vi "DIO64 Sequence.vi"(0 "DIO64Addr (0)":u16, 1 "RepRate (Hz)":dbl, 3 "Config Control":T1={"flags"=enum."unused", "clock control"=enum."external", "start trigger"={"source"=enum."external", "type"=enum."edge", "sense"=enum."rising"}, "stop trigger"={"source"=enum."output FIFO", "type"=enum."level", "sense"=enum."falling"}, "DAQ clock modulo"=0, "repetitions"=0, "#transitions"=0} {"#transitions" format="%.0x"; "repetitions" format="%.0x"; "DAQ clock modulo" format="%.0x"}, 5 "Time Array (ms)":dbl[](array[numeric])=[0.0, 1.0, 2.1658, 2.4158, 2.5658, 2.5757999999999996, 2.7057999999999995, 2.7157999999999993, 3.1699999999999995, 3.1913999999999993, 3.2021999999999995, 3.2031999999999994, 3.2226999999999992, 3.223699999999999, 4.223699999999999] caption="Time of step .. (ms)", 7 "Set DIO line ..":bool[][](array[boolean])=[[FALSE, FALSE, FALSE, FALSE, FALSE, FALSE, FALSE, FALSE, FALSE, FALSE, FALSE, FALSE, FALSE, FALSE, FALSE, FALSE], [FALSE, FALSE, FALSE, FALSE, FALSE, FALSE, FALSE, FALSE, FALSE, FALSE, FALSE, FALSE, FALSE, FALSE, FALSE, FALSE], [FALSE, FALSE, FALSE, FALSE, FALSE, FALSE, TRUE, FALSE, FALSE, FALSE, FALSE, FALSE, FALSE, FALSE, FALSE, FALSE], [FALSE, FALSE, FALSE, FALSE, FALSE, FALSE, FALSE, FALSE, FALSE, FALSE, FALSE, FALSE, FALSE, FALSE, FALSE, FALSE], [FALSE, FALSE, FALSE, FALSE, TRUE, FALSE, FALSE, FALSE, FALSE, FALSE, FALSE, FALSE, FALSE, FALSE, FALSE, FALSE], [FALSE, FALSE, FALSE, FALSE, FALSE, FALSE, FALSE, FALSE, FALSE, FALSE, FALSE, FALSE, FALSE, FALSE, FALSE, FALSE], [FALSE, FALSE, FALSE, FALSE, FALSE, TRUE, FALSE, FALSE, FALSE, FALSE, FALSE, FALSE, FALSE, FALSE, FALSE, FALSE], [FALSE, FALSE, FALSE, FALSE, FALSE, FALSE, FALSE, FALSE, FALSE, FALSE, FALSE, FALSE, FALSE, FALSE, FALSE, FALSE], [FALSE, FALSE, FALSE, FALSE, FALSE, FALSE, FALSE, FALSE, FALSE, TRUE, FALSE, FALSE, FALSE, FALSE, FALSE, FALSE], [FALSE, FALSE, FALSE, FALSE, FALSE, FALSE, FALSE, FALSE, FALSE, FALSE, TRUE, FALSE, FALSE, FALSE, FALSE, FALSE], [FALSE, FALSE, FALSE, TRUE, FALSE, FALSE, FALSE, FALSE, FALSE, FALSE, FALSE, FALSE, FALSE, FALSE, FALSE, FALSE], [FALSE, FALSE, FALSE, FALSE, FALSE, FALSE, FALSE, FALSE, FALSE, FALSE, FALSE, FALSE, FALSE, FALSE, FALSE, FALSE], [FALSE, FALSE, FALSE, FALSE, FALSE, FALSE, FALSE, TRUE, FALSE, FALSE, FALSE, FALSE, FALSE, FALSE, FALSE, FALSE], [FALSE, FALSE, FALSE, FALSE, FALSE, FALSE, FALSE, FALSE, FALSE, FALSE, FALSE, FALSE, FALSE, FALSE, FALSE, FALSE]] caption="Set DIO lines in step ..", 9 "output cluster":cluster{bool[][], bool[][], bool[][], bool[][]}, 11 "error in":errorcluster={"status"=FALSE, "code"=0, "source"="DIO64 Out Stop"}) -> (15 "error out":errorcluster={"status"=FALSE, "code"=0, "source"="DIO64 Out Stop"})   [LabVIEW 2012]
doc: "Sets the DIO-Board to - \"Continous Mode\" and\n - External Triggering (Edge, rising)\n(the Default values of the ConfigControl are set accordingly)\n\nand waits for a time of 1/RepRate * #Shots\n or Time of Sequence * #Shots,\nwhichever is larger (+100 ms).\nThe DIO-Board is then stopped."
uses:
  DIO64 Out Config Control.ctl
  DIO64 Clock Control.ctl
  DIO64 Start Trig.ctl
  DIO64 Stop Trig.ctl
  DIO64 attribute id.ctl
  DIO64 attribute value.ctl
panel:
  out "stop time":u32 format="%.6f"
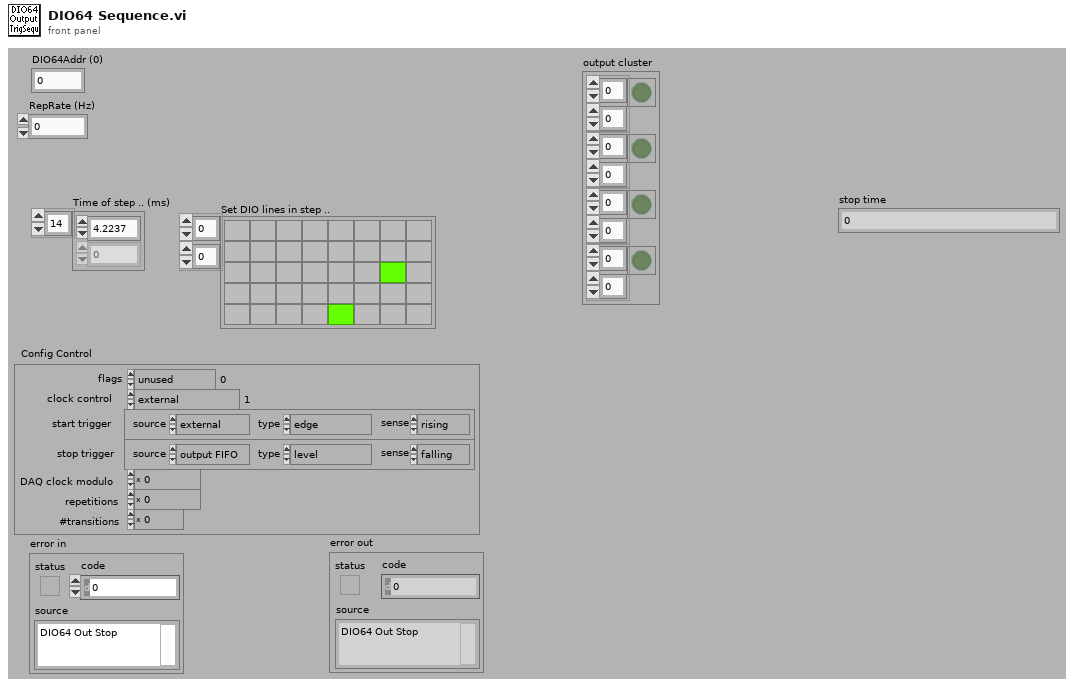
[diagram p1: front panel]
types:
  T1 = typedef "DIO64 Out Config Control.ctl" = cluster{"flags":enum16{"unused"}, "clock control":T2, "start trigger":T3, "stop trigger":T4, "DAQ clock modulo":u32, "repetitions":u32, "#transitions":u16}
  T2 = typedef "DIO64 Clock Control.ctl" = enum16{"internal", "external", "trig 0", "OCXO"}
  T3 = typedef "DIO64 Start Trig.ctl" = cluster{"source":enum16{"none", "internal", "external", "trig 2", "PXI Star"}, "type":enum16{"level", "edge", "edge to edge"}, "sense":enum16{"rising", "falling"}}
  T4 = typedef "DIO64 Stop Trig.ctl" = cluster{"source":enum16{"none", "internal", "external", "trig 3 in", "output FIFO"}, "type":enum16{"level", "edge"}, "sense":enum16{"falling", "rising"}}
  T5 = enum32{"invalid OS target", "Mac OS", "Windows 3.1", "Windows 95/NT", "Solaris 1", "Solaris 2", "HP-UX", "PowerMAX", "Linux", "Irix", "Rhapsody", "BeOS", "AIX", "OSF1", "VxWorks", "PharLap", "Carbon", "RTX", "Windows x64", "Linux x64"}
  T6 = typedef "DIO64 attribute value.ctl" = enum16{"default", "long value", "polled", "interrupt", "packet", "demand", "local clock", "external clock", "rtsi/pxi clock", "precision clock", "20MHz", "10MHz", "precision OCXO", "enable", "disable"}
  T7 = typedef "DIO64 attribute id.ctl" = enum16{"input mode", "output mode", "input buffer size", "output buffer size", "major clock source", "input threshold percent", "output threshold percent", "input dma timeout", "rtsi/pxi global enable", "rtsi/pxi clock source", "rtsi clock/pxi trig 7 enable", "external clock enable", "pxi clock enable", "scan clock trig 0 enable", "start trig trig 2 enable", "stop trig trig 3 enable", "daq modulo trig 4 enable", "pxi star enable", "port routing", "staticOutputPorts", "serial number"}
  T8 = typedef "DIO64 Out Status.ctl" = cluster{"pktsize":u16, "portCount":u16, "writePtr":u16, "readPtr":u16, "time0":u16, "time1":u16, "fifoSize":u32, "fifo0":u16, "ticks":u32, "flags":u16, "clkControl":u16, "startControl":u16, "stopControl":u16, "AIControl":u32, "AICurrent":u16, "startTime0":u16, "startTime1":u16, "stopTime0":u16, "stopTime1":u16, "#trans":u16, "reps":u16, "cur trans":u16, "cur reps":u16}
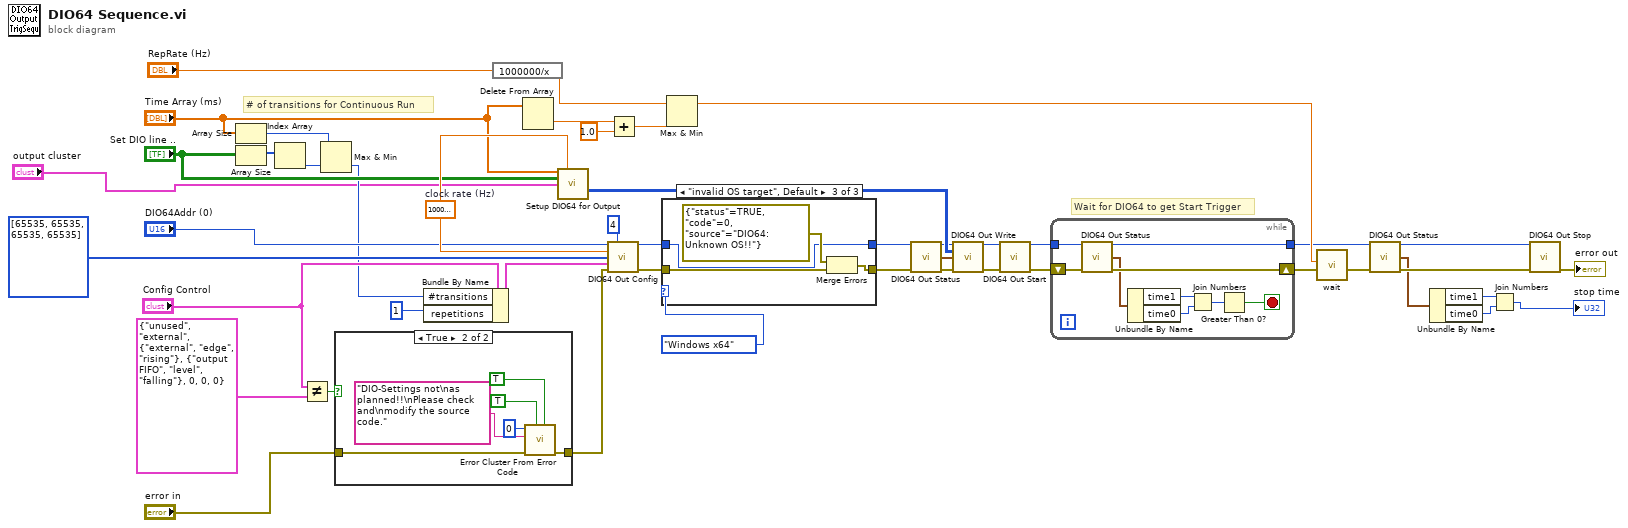
[diagram p0: block diagram]
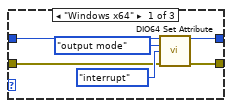
[diagram p2: hidden frame]
diagram:
  w47 = 10000000.0  # clock rate (Hz)
  # "Wait for DIO64 to get Start Trigger"
  # "# of transitions for Continuous Run"
  n1 = Array Size(array="Time Array (ms)") -> (size(s)=w38:i32)
  n2 = Array Size(array="Set DIO line ..") -> (size(s)=w40:i32[])
  n3 = Index Array(array=w40) -> (element=w39:i32)  [unwired: 1 in]
  n4 = Not Equal?(x="Config Control", y=T1 {"flags"=enum."unused", "clock control"=enum."external", "start trigger"={"source"=enum."external", "type"=enum."edge", "sense"=enum."rising"}, "stop trigger"={"source"=enum."output FIFO", "type"=enum."level", "sense"=enum."falling"}, "DAQ clock modulo"=0, "repetitions"=0, "#transitions"=0} ("Config Control 2")) -> (x != y?=w43:bool)
  n5 = Max & Min(x=w38, y=w39) -> (min(x,y)=w36:i32)  [unwired: 1 out]
  n6 = case shown="True" w43 {
    tunnel: "error in" -> [w48 w54]
    tunnel: [w48 w50] -> w23
    frame False {
    }
    frame True {
      n7 = call <vilib>:"Error Cluster From Error Code.vi"("is warning? (False)"=TRUE, "show call chain? (False)"=TRUE, "error in (no error)"=w54, "error message (\"\")"="DIO-Settings not\nas planned!!\nPlease check and\nmodify the source code.", "error code (0)"=0) -> ("error out"=w50:errorcluster)  [unwired: 4 in]
    }
  }
  n8 = Bundle By Name(cluster="Config Control", "#transitions"=w36, "repetitions"=u32 1) -> (w35:T1)
  n9 = expression code="1000000/x"("RepRate (Hz)") -> (w32:dbl)
  n10 = Delete From Array(array="Time Array (ms)") -> (deleted portion=w20:dbl)  [unwired: 2 in, 1 out]
  n11 = call "Setup DIO64 for Output.vi"("timestamps (ms)"="Time Array (ms)", "scan rate (Hz)"=w47, "bitmap"="Set DIO line ..", "output cluster"="output cluster") -> ("data"=w33:u16[][])  [unwired: 11 in]
  n12 = call "DIO64 Out Config.vi"("board in"="DIO64Addr (0)", "#ports"=u8 4, "scan rate (Hz)"=w47, "mask"=u16[] [65535, 65535, 65535, 65535], "Config Control"=w35, "error in (no error)"=w23) -> ("board out"=w14:u16, "error out"=w16:errorcluster)  [unwired: 7 in, 1 out]
  n13 = Add(x=w20, y=1.0) -> (x+y=w19:dbl)
  n14 = case shown="\"invalid OS target\", Default" T5."Windows x64" ("App.TargetOS") {
    tunnel: [w58 w62 w65] -> w15
    tunnel: w16 -> [w57 w62 w66]
    tunnel: w14 -> [w56 w61 w63]
    tunnel: [w55 w61 w63] -> w13
    frame "Windows x64" {
      n15 = call "DIO64 Set Attribute.vi"("board in"=w56, "attribute id"=DIO64_attribute_id."output mode", "attribute value"=DIO64_attribute_value."interrupt", "error in (no error)"=w57) -> ("board out"=w55:u16, "error out"=w58:errorcluster)  [unwired: 10 in]
    }
    frame "Windows 95/NT" {
    }
    frame "invalid OS target", Default {
      n16 = Merge Errors(errorcluster {"status"=TRUE, "code"=0, "source"="DIO64: Unknown OS!!"} ("error constant"), w66) -> (w65:errorcluster)
    }
  }
  n17 = Max & Min(x=w32, y=w19) -> (max(x,y)=w21:dbl)  [unwired: 1 out]
  n18 = call "DIO64 Out Status.vi"("board in"=w13, "error in (no error)"=w15) -> ("board out"=w27:u16, "Out Status"=w29:T8, "error out"=w28:errorcluster)  [unwired: 10 in, 1 out]
  n19 = call "DIO64 Out Write.vi"("board in"=w27, "data"=w33, "Out Status"=w29, "error in (no error)"=w28) -> ("board out"=w26:u16, "error out"=w25:errorcluster)  [unwired: 10 in]
  n20 = call "DIO64 Out Start.vi"("board in"=w26, "error in (no error)"=w25) -> ("board out"=w10:u16, "error out"=w11:errorcluster)  [unwired: 12 in]
  n21 = while {
    tunnel: w10 -> [w74]
    tunnel: [w72] -> w6
    shift-right: [w73] -> w9
    shift-left: w11 -> [w75]
    stop <- w67 stop-if-true
    n22 = call "DIO64 Out Status.vi"("board in"=w74, "error in (no error)"=w75) -> ("board out"=w72:u16, "Out Status"=w71:T8, "error out"=w73:errorcluster)  [unwired: 10 in, 1 out]
    n23 = Unbundle By Name(w71) -> ("time1"=w70:u16, "time0"=w69:u16)
    n24 = Join Numbers(hi=w70, lo=w69) -> ((hi.lo)=w68:u32)
    n25 = Greater Than 0?(x=w68) -> (x > 0?=w67:bool)
  }
  n26 = call "wait.vi"("error in (no error)"=w9, "ms to wait"=w21) -> ("error out (no error)"=w8:errorcluster)  [unwired: 7 in]
  n27 = call "DIO64 Out Status.vi"("board in"=w6, "error in (no error)"=w8) -> ("board out"=w5:u16, "Out Status"=w2:T8, "error out"=w7:errorcluster)  [unwired: 10 in, 1 out]
  n28 = Unbundle By Name(w2) -> ("time1"=w3:u16, "time0"=w4:u16)
  n29 = Join Numbers(hi=w3, lo=w4) -> ((hi.lo)=→"stop time":u32)
  n30 = call "DIO64 Out Stop.vi"("board in"=w5, "error in (no error)"=w7) -> ("error out"=→"error out":errorcluster)  [unwired: 12 in, 1 out]
